vi "Draw Y=0 Line.vi"(6 "Needs update":bool, 8 "error in (no error)":errorcluster, 9 "PreviewGraph Ref":refnum<vi>, 10 "Data In":T1 caption="Waveform Data", 11 "Display State In":T2={"Show Axes"=FALSE, "Show Y=0"=FALSE, "Controls"={"Type"=enum."Sine", "Periods"=0.0, "Points"=0, "Offset"=0.0, "Amplitdue"=0.0, "Starting Phase"=0.0, "func"=""}, "Show Current Location"=FALSE, "Current Location"=0, "dt"=0.0, "t0"=timestamp(0 s since 1904-01-01), "Amplitude Format String"="%_3p"} caption="State" {"Controls"."Points" format="%_3p"}) -> (0 "error ou":errorcluster, 3 "Display State Out":T2={"Show Axes"=FALSE, "Show Y=0"=FALSE, "Controls"={"Type"=enum."Sine", "Periods"=0.0, "Points"=0, "Offset"=0.0, "Amplitdue"=0.0, "Starting Phase"=0.0, "func"=""}, "Show Current Location"=FALSE, "Current Location"=0, "dt"=0.0, "t0"=timestamp(0 s since 1904-01-01), "Amplitude Format String"="%_3p"} caption="State" {"Controls"."Points" format="%_3p"})   [LabVIEW 2018, in "Waveform Control.xctl"]
uses:
  Waveform Control.xctl
  Controls/Waveform State.ctl
  FP Controls.ctl
  Function Types.ctl
  Controls/Data.ctl
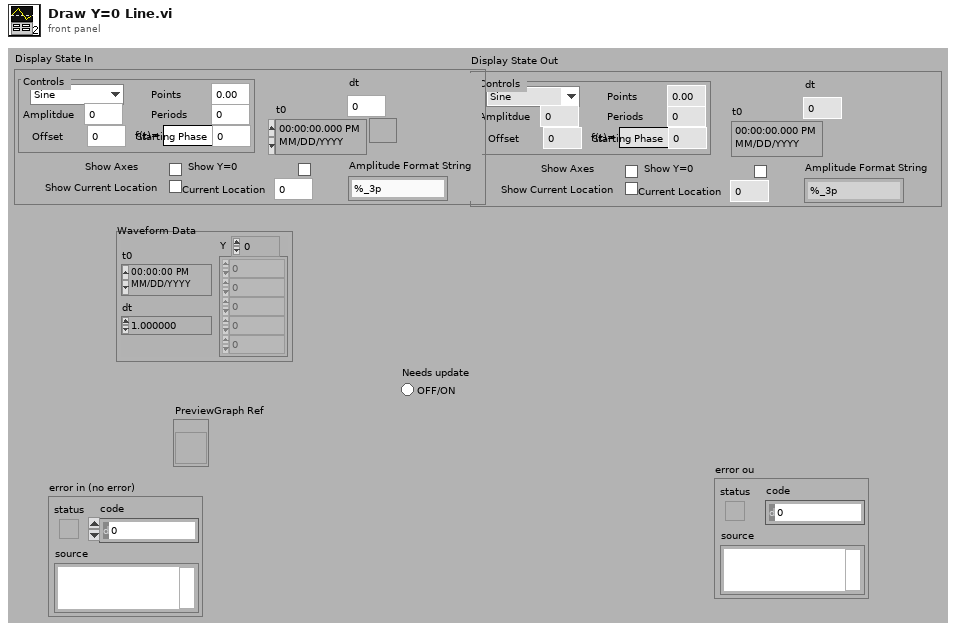
[diagram p1: front panel]
types:
  T1 = typedef "Waveform Control.xctl/Data.ctl" = waveform(dbl)
  T2 = typedef "Waveform Control.xctl/Waveform State.ctl" = cluster{"Show Axes":bool, "Show Y=0":bool, "Controls":T3, "Show Current Location":bool, "Current Location":i32, "dt":dbl, "t0":timestamp, "Amplitude Format String":string}
  T3 = typedef "Waveform Control.xctl/FP Controls.ctl" = cluster{"Type":T4, "Periods":dbl, "Points":i32, "Offset":dbl, "Amplitdue":dbl, "Starting Phase":dbl, "func":string}
  T4 = typedef "Waveform Control.xctl/Function Types.ctl" = enum16{"Level", "Sine", "Triangle", "Ramp", "Saw Tooth", "Square", "Function"}
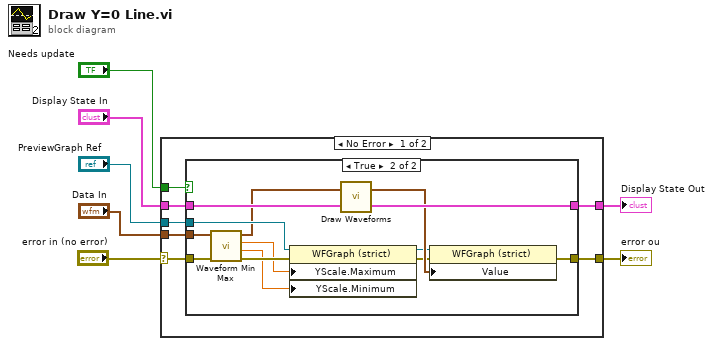
[diagram p0: block diagram]
diagram:
  n1 = case shown="No Error" "error in (no error)" {
    selector: "error in (no error)" -> [w13 w31]
    tunnel: [w14 w31] -> w7
    tunnel: [w12 w30] -> w5
    tunnel: "Data In" -> [w11 _]
    tunnel: "PreviewGraph Ref" -> [w10 _]
    tunnel: "Display State In" -> [w9 w30]
    tunnel: "Needs update" -> [w8 _]
    frame No Error {
      n2 = case shown="True" w8 {
        tunnel: w11 -> [_ w29]
        tunnel: w9 -> [w16 w28]
        tunnel: [w16 w27] -> w12
        tunnel: w13 -> [w15 w22]
        tunnel: [w15 w25] -> w14
        tunnel: w10 -> [_ w24]
        frame False {
        }
        frame True {
          n3 = call <vilib>:"Waveform Min Max.vi"("error in (no error)"=w22, "waveform in"=w29) -> ("error out"=w20:errorcluster, "Y min"=w17:dbl, "Y max"=w18:dbl, "waveform out"=w23:waveform(dbl))  [unwired: 6 out]
          n4 = property class="WFGraph (strict)"(reference=w24, error in=w20, "YScale.Maximum"=w18, "YScale.Minimum"=w17) -> (reference out=w21:refnum<vi>, error out=w19:errorcluster)
          n5 = call "Draw Waveforms.vi"("Display State In"=w28, "Data In"=w23) -> ("Display State Out"=w27:T2, "Array"=w26:T1[])
          n6 = property on="Property Node" class="WFGraph (strict)"(reference=w21, error in=w19, "Value"=w26) -> (error out=w25:errorcluster)  [unwired: 1 out]
        }
      }
    }
    frame Error {
    }
  }
  "error ou" <- w7
  "Display State Out" <- w5
